vi "LVClass_HasoData Apply Slopes Processor List.vi"(0 "HasoData in":refnum<class "HasoData.lvclass">, 5 "SlopesPostProcessorList":refnum<class "SlopesPostProcessorList.lvclass">, 11 "error in (no error)":errorcluster) -> (4 "HasoData out":refnum<class "HasoData.lvclass">, 15 "error out":errorcluster)   [LabVIEW 2020, in "HasoData.lvclass"]
doc: "Apply a SlopesPostProcessorList to the raw HasoSlopes stores in the HasoData\nobject.\n\n--------------------------------------------------------------------------------\n\n<B>HasoDataIn </B> : HasoData object.\n<B>HasoDataOut </B> : HasoData object.\n<B>SlopesPostProcessorList </B> : SlopesPostProcessorList object.\n<B>ErrorIn </B> : Error\n<B>ErrorOut </B> : Error\n\n--------------------------------------------------------------------------------"
uses:
  HasoData.lvclass
  SlopesPostProcessorList.lvclass
  HasoData.lvclass/HasoData.ctl
  LVClass_SlopesPostProcessList Read SlopesPostProccessor.vi
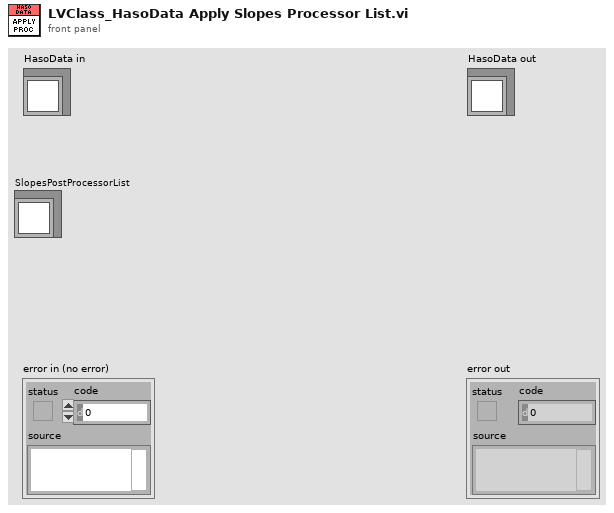
[diagram p1: front panel]
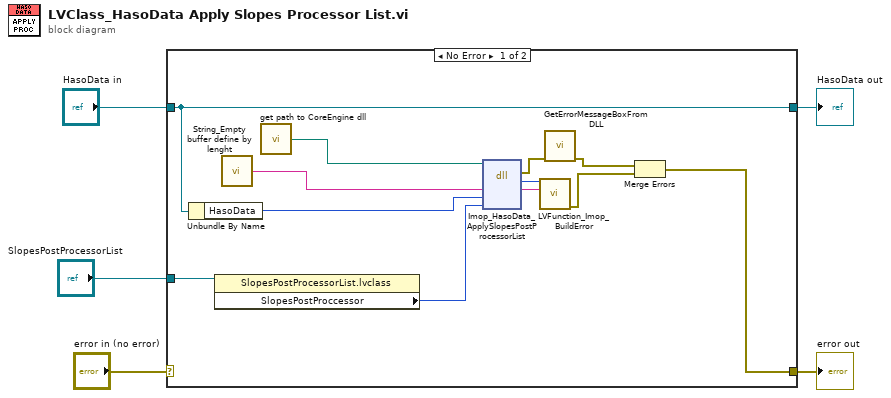
[diagram p0: block diagram]
diagram:
  n1 = case shown="No Error" "error in (no error)" {
    selector: "error in (no error)" -> [_ w19]
    tunnel: [w6 w19] -> w3
    tunnel: [w13 w18] -> w2
    tunnel: "HasoData in" -> [w13 w18]
    tunnel: "SlopesPostProcessorList" -> [w10 _]
    frame No Error {
      n2 = Unbundle By Name(w13) -> ("HasoData"=w14:i32)
      n3 = property class="SlopesPostProcessorList.lvclass"(reference=w10) -> ("SlopesPostProccessor"=w9:i32)  [unwired: 1 in, 2 out]
      n4 = call "String_Empty buffer define by lenght.vi"() -> ("Empty buffer"=w15:string)  [unwired: 1 in]
      n5 = call "get path to CoreEngine dll.vi"() -> ("path to c_interface_vc100.dll"=w12:path)  [unwired: 12 in, 3 out]
      n6 = dll-call lib="D:/2_trunk/Soft_haso/ImOpCoreEngine4_LV2011/DLLs/ImopEngine4_vc100.dll" fn="Imop_HasoData_ApplySlopesPostProcessorList"(path in=w12, "message"=w15, "objet"=w14, "Slopes_Post_Process_List"=w9) -> (error out=w11:errorcluster, "return type"=w17:i32, "message"=w16:string)  [unwired: 4 in, 1 out]
      n7 = call "LVFunction_Imop_BuildError.vi"("code"=w17, "String to Prepend to source (\"\")"=w16) -> ("error out"=w7:errorcluster)  [unwired: 13 in]
      n8 = call "GetErrorMessageBoxFromDLL.vi"("error IN"=w11) -> ("error OUT"=w8:errorcluster)  [unwired: 10 in]
      n9 = Merge Errors(w8, w7) -> (w6:errorcluster)
    }
    frame Error {
    }
  }
  "error out" <- w3
  "HasoData out" <- w2
